vi "Read Constants.vi"(8 "error in (no error)":errorcluster, 11 "mupExpr in":refnum<class "mupExpr.lvclass">) -> (0 "error out":errorcluster, 2 "Constants":cluster{"name":string, "value":dbl}[](array[cluster]), 3 "mupExpr out":refnum<class "mupExpr.lvclass">)   [LabVIEW 2015, in "mupExpr.lvclass"]
uses:
  mupExpr.lvclass
  mupExpr.lvclass/mupExpr.ctl
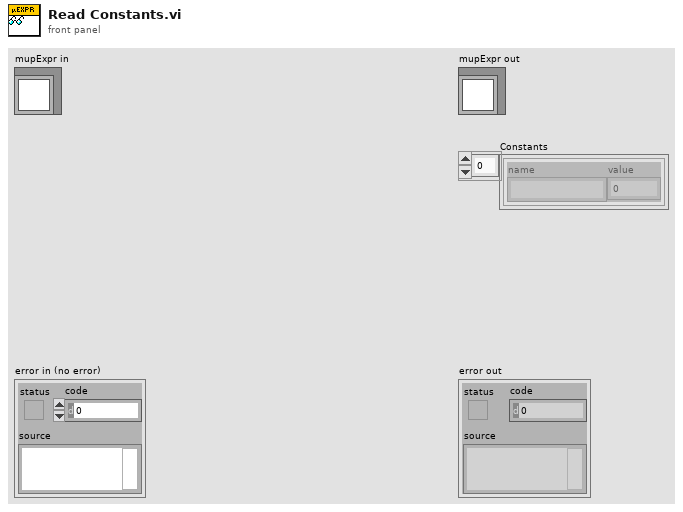
[diagram p1: front panel]
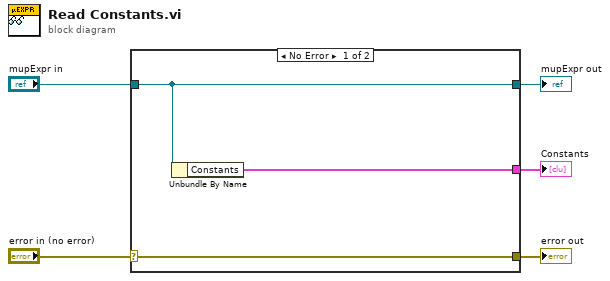
[diagram p0: block diagram]
diagram:
  n1 = case shown="No Error" "error in (no error)" {
    selector: "error in (no error)" -> [w8 w9]
    tunnel: [w8 w9] -> w4
    tunnel: [w7 w10] -> w2
    tunnel: "mupExpr in" -> [w7 w10]
    tunnel: [w6 _] -> w1
    frame No Error {
      n2 = Unbundle By Name(w7) -> ("Constants"=w6:cluster{"name":string, "value":dbl}[])
    }
    frame Error {
    }
  }
  "error out" <- w4
  "mupExpr out" <- w2
  "Constants" <- w1
